vi "motionProfileTelemetry.vi"(9 "Pigeon":T2={"DeviceStatus"={"status"=FALSE, "code"=0, "source"=""}, "Device Number"=0, "Type"=352321536, "Device ID"=0, "Handle"=0, "UsageFrame"=0, "Library Path"=path ""} {"Type" items=["CAN"=352321536, "TalonSRX"=33554432]}, 10 "Alt Talon":T4={"DeviceStatus"={"status"=FALSE, "code"=0, "source"=""}, "Type"=enum."PWM", "PWM"={"PWM Channel"=enum."Invalid", "DeadBand"={"Name"="", "maxPositivePwm"=0, "minPositivePwm"=0, "centerPwm"=0, "maxNegativePwm"=0, "minNegativePwm"=0, "angularRange"=0}}, "CAN"={"Device Number"=0, "SetOutput VI Ref"=variant, "GetOutput VI Ref"=variant, "Enable VI Ref"=variant, "Disable VI Ref"=variant, "Data"=variant}, "Invert"=FALSE, "DIO PWM"={"PWM \"Enable\" Channel"=enum."Invalid", "DIOChannel"=enum."Invalid", "PWM Rate"=0.0}}, 11 "Main Talon":T4={"DeviceStatus"={"status"=FALSE, "code"=0, "source"=""}, "Type"=enum."PWM", "PWM"={"PWM Channel"=enum."Invalid", "DeadBand"={"Name"="", "maxPositivePwm"=0, "minPositivePwm"=0, "centerPwm"=0, "maxNegativePwm"=0, "minNegativePwm"=0, "angularRange"=0}}, "CAN"={"Device Number"=0, "SetOutput VI Ref"=variant, "GetOutput VI Ref"=variant, "Enable VI Ref"=variant, "Disable VI Ref"=variant, "Data"=variant}, "Invert"=FALSE, "DIO PWM"={"PWM \"Enable\" Channel"=enum."Invalid", "DIOChannel"=enum."Invalid", "PWM Rate"=0.0}}) -> ()   [LabVIEW 2018]
uses:
  <vilib>/Rock Robotics/WPI/MotorControl/WPI_MotorControlDeviceRef.ctl
  <vilib>/Rock Robotics/WPI/MotorControl/WPI_MotorControlType.ctl
  <vilib>/Rock Robotics/SystemInterfaces/DIO/FPGA_DIOPWMChannel.ctl
  <vilib>/Rock Robotics/WPI/PWM/WPI_PWMDeadband.ctl
  <vilib>/Rock Robotics/SystemInterfaces/DIO/FPGA_DIOChannel.ctl
  <vilib>/Rock Robotics/WPI/ThirdParty/Phoenix-LabVIEW/Pigeon IMU/CTRE_PigeonIMU_DeviceRef.ctl
  <vilib>/Rock Robotics/WPI/ThirdParty/Phoenix-LabVIEW/Pigeon IMU/CTRE_PigeonIMU_ConnectionType.ctl
  driveShifterEnum.ctl
  <vilib>/Rock Robotics/WPI/ThirdParty/Phoenix-LabVIEW/Pigeon IMU/CTRE_PigeonIMU_CalibrationMode.ctl
  <vilib>/Rock Robotics/WPI/ThirdParty/Phoenix-LabVIEW/Motor Controller/Get/CTRE_Phoenix_MotorController_GetVoltage.vi
  <vilib>/Rock Robotics/WPI/ThirdParty/Phoenix-LabVIEW/Motor Controller/Get/CTRE_Phoenix_MotorController_GetQuadratureData.vi
panel:
  out "driveIMUYawPitchRoll":cluster{"Yaw":dbl, "Pitch":dbl, "Roll":dbl}
  out "driveFusedHeading":T1
  in  "Calibrate IMU":bool
  in  "Reset PID":bool
  out "Percent Out":T9(graph)
  out "Motion Profile Status":T10
  out "Turn":cluster{dbl, "x-y":dbl}[](graph)
  out "Position":cluster{"x-y":dbl, i32}[](graph)
  out "Velocity":cluster{"Output":dbl, "Double":dbl}[](graph)
  out "Right Velocity":i32
  out "Right Position":i32=-2624
  out "Left Velocity":i32
  out "Left Position":i32=2620
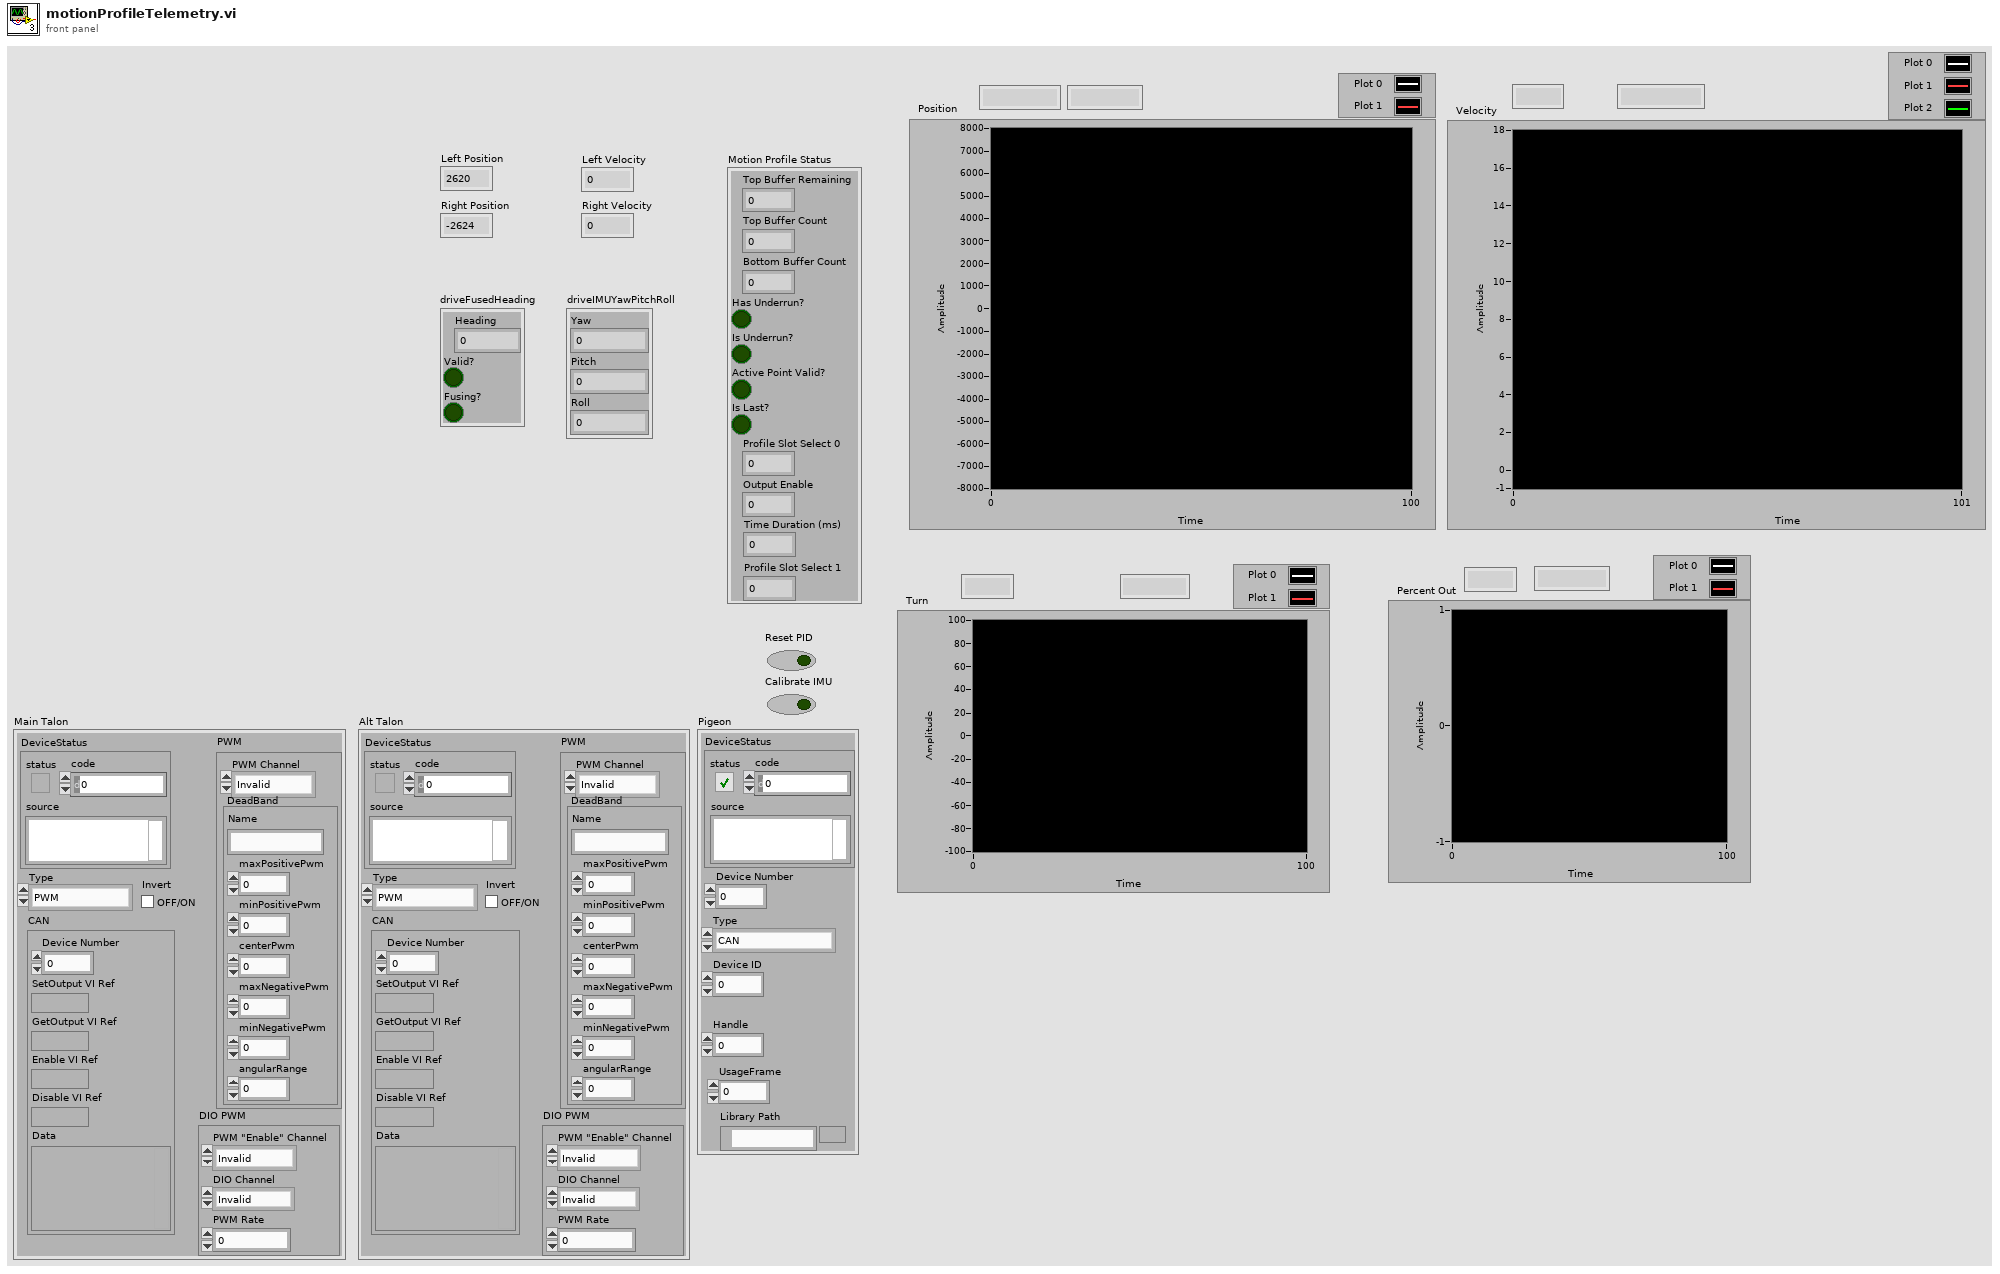
[diagram p1: front panel]
types:
  T1 = cluster{"Heading":dbl, "Valid?":bool, "Fusing?":bool}
  T2 = typedef "CTRE_PigeonIMU_DeviceRef.ctl" = cluster{"DeviceStatus":errorcluster, "Device Number":u8, "Type":T3, "Device ID":u32, "Handle":u64, "UsageFrame":u32, "Library Path":path}
  T3 = typedef "CTRE_PigeonIMU_ConnectionType.ctl" = u32
  T4 = typedef "WPI_MotorControlDeviceRef.ctl" = cluster{"DeviceStatus":errorcluster, "Type":T5, "PWM":cluster{"PWM Channel":T6, "DeadBand":T7}, "CAN":cluster{"Device Number":u8, "SetOutput VI Ref":variant, "GetOutput VI Ref":variant, "Enable VI Ref":variant, "Disable VI Ref":variant, "Data":variant}, "Invert":bool, "DIO PWM":cluster{"PWM \"Enable\" Channel":T6, "DIOChannel":T8, "PWM Rate":dbl}}
  T5 = typedef "WPI_MotorControlType.ctl" = enum16{"PWM", "CAN", "DIO PWM"}
  T6 = typedef "FPGA_DIOPWMChannel.ctl" = enum8{"PWM 0", "PWM 1", "PWM 2", "PWM 3", "PWM 4", "PWM 5", "PWM 6", "PWM 7", "PWM 8", "PWM 9", "PWM MXP 0", "PWM MXP 1", "PWM MXP 2", "PWM MXP 3", "PWM MXP 4", "PWM MXP 5", "PWM MXP 6", "PWM MXP 7", "PWM MXP 8", "PWM MXP 9", "Invalid"}
  T7 = typedef "WPI_PWMDeadband.ctl" = cluster{"Name":string, "maxPositivePwm":i32, "minPositivePwm":i32, "centerPwm":i32, "maxNegativePwm":i32, "minNegativePwm":i32, "angularRange":u16}
  T8 = typedef "FPGA_DIOChannel.ctl" = enum8{"DIO 0", "DIO 1", "DIO 2", "DIO 3", "DIO 4", "DIO 5", "DIO 6", "DIO 7", "DIO 8", "DIO 9", "DIO MXP 0", "DIO MXP 1", "DIO MXP 2", "DIO MXP 3", "DIO MXP 4", "DIO MXP 5", "DIO MXP 6", "DIO MXP 7", "DIO MXP 8", "DIO MXP 9", "DIO MXP 10", "DIO MXP 11", "DIO MXP 12", "DIO MXP 13", "DIO MXP 14", "DIO MXP 15", "SPI Port CS1", "SPI Port CS2", "SPI Port CS3", "SPI Port MISO", "SPI Port MOSI", "Invalid"}
  T9 = cluster{"Percent Output":dbl, "Percent Output":dbl}[]
  T10 = cluster{"Top Buffer Remaining":i32, "Top Buffer Count":i32, "Bottom Buffer Count":i32, "Has Underrun?":bool, "Is Underrun?":bool, "Active Point Valid?":bool, "Is Last?":bool, "Profile Slot Select 0":i32, "Output Enable":i32, "Time Duration (ms)":i32, "Profile Slot Select 1":i32}
  T11 = typedef "driveShifterEnum.ctl" = enum16{"Low", "High"}
  T12 = enum16{"Inches -> Sensor Units", "Sensor Units -> Inches"}
  T13 = typedef "CTRE_PigeonIMU_CalibrationMode.ctl" = u16
  T14 = cluster{"Percent Output":dbl, "Percent Output":dbl}
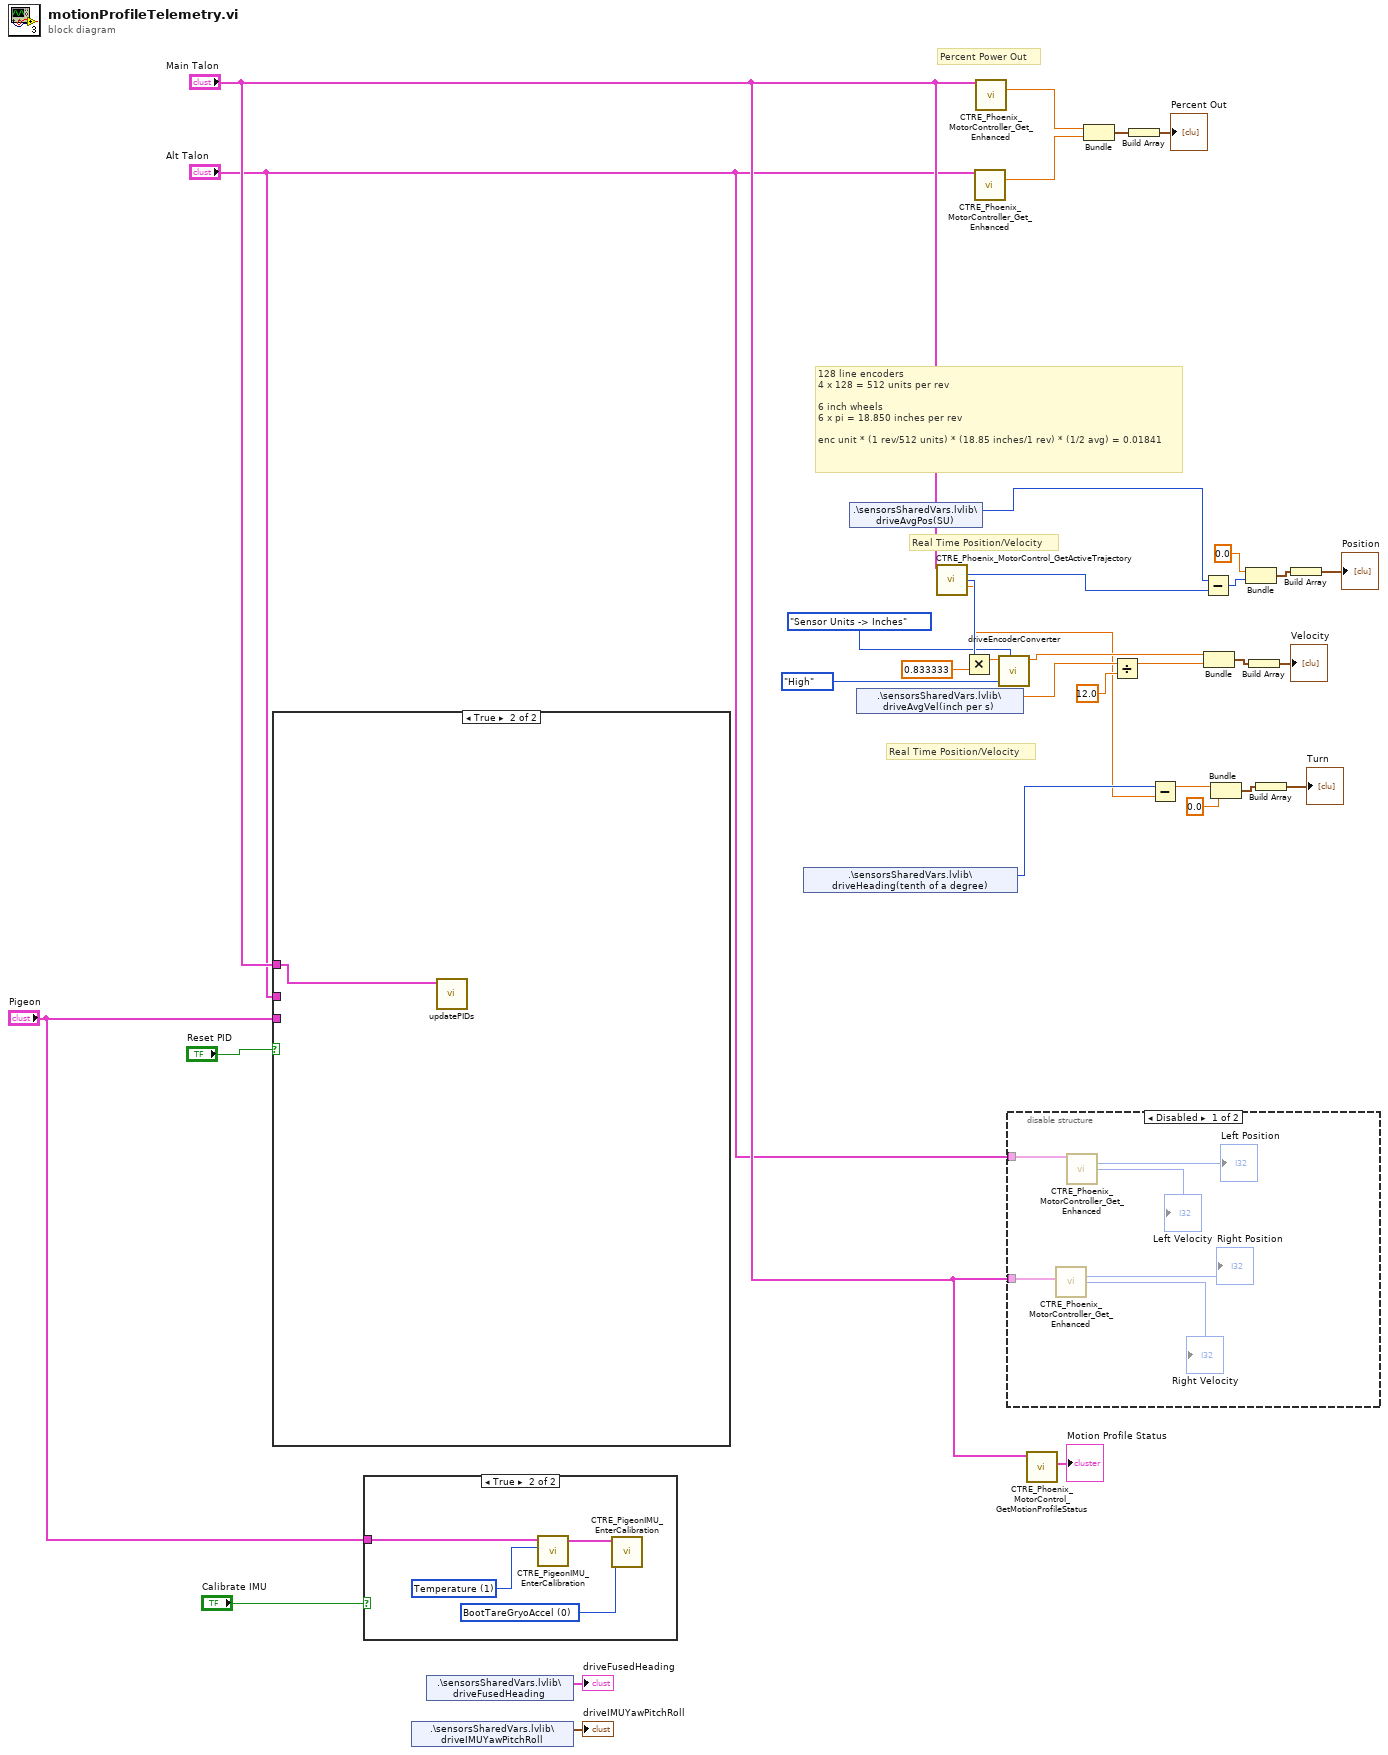
[diagram p0: block diagram]
diagram:
  # "Percent Power Out"
  # "Real Time Position/Velocity"
  # "Real Time Position/Velocity"
  # "128 line encoders\n4 x 128 = 512 units per rev\n\n6 inch wheels\n6 x pi = 18.850 inches per rev\n\nenc unit * (1 rev/512 units) * (18.85 inches/1 rev) * (1/2 avg) = 0.01841"
  n1 = case shown="True" "Reset PID" {
    tunnel: "Main Talon" -> [_ w36]
    tunnel: "Alt Talon" -> [_ _]
    tunnel: "Pigeon" -> [_ _]
    frame False {
    }
    frame True {
      n2 = call "updatePIDs.vi"("MainTalon"=w36) -> ()  [unwired: 11 in]
    }
  }
  n3 = case shown="True" "Calibrate IMU" {
    tunnel: "Pigeon" -> [_ w40]
    frame False {
    }
    frame True {
      w37 = T13 0 items=["BootTareGryoAccel"=0, "Temperature"=1, "Magnetometer12Pt"=2, "Magnetometer360"=3, "Accelerometer"=5] ("CalibrationMode")
      w39 = T13 1 items=["BootTareGryoAccel"=0, "Temperature"=1, "Magnetometer12Pt"=2, "Magnetometer360"=3, "Accelerometer"=5] ("CalibrationMode")
      n4 = call <vilib>:"CTRE_PigeonIMU_EnterCalibration.vi"("CalibrationMode"=w39, "PigeonIMUDevRef"=w40) -> ("PigeonIMUDevRef"=w38:T2)  [unwired: 8 in, 1 out]
      n5 = call <vilib>:"CTRE_PigeonIMU_EnterCalibration.vi"("CalibrationMode"=w37, "PigeonIMUDevRef"=w38) -> ()  [unwired: 8 in, 2 out]
    }
  }
  n6 = shared-variable ".\\sensorsSharedVars.lvlib\\driveIMUYawPitchRoll"() -> (→"driveIMUYawPitchRoll":cluster{"Yaw":dbl, "Pitch":dbl, "Roll":dbl})  [unwired: 1 in, 1 out]
  n7 = shared-variable ".\\sensorsSharedVars.lvlib\\driveFusedHeading"() -> (→"driveFusedHeading":T1)  [unwired: 1 in, 1 out]
  n8 = shared-variable ".\\sensorsSharedVars.lvlib\\driveHeading(tenth of a degree)"() -> (w25:i32)  [unwired: 1 in, 1 out]
  n9 = shared-variable ".\\sensorsSharedVars.lvlib\\driveAvgPos(SU)"() -> (w13:i32)  [unwired: 1 in, 1 out]
  n10 = shared-variable ".\\sensorsSharedVars.lvlib\\driveAvgVel(inch per s)"() -> (w23:dbl)  [unwired: 1 in, 1 out]
  n11 = call <vilib>:"CTRE_Phoenix_MotorControl_GetActiveTrajectory.vi"("PhoenixMotorControlDevRef"="Main Talon") -> ("Position (Sensor Units)"=w11:i32, "Velocity (Sensor Units per 100 ms)"=w22:i32, "Heading"=w9:dbl)  [unwired: 10 in, 2 out]
  n12 = Multiply(x=w22, y=0.833333) -> (x*y=w19:dbl)
  n13 = call-poly <vilib>:"CTRE_Phoenix_MotorController_Get_Enhanced.vi"("PhoenixMotorControlDevRef"="Alt Talon") -> ("Percent Output"=w2:dbl)  [unwired: 10 in, 4 out]
  n14 = call-poly <vilib>:"CTRE_Phoenix_MotorController_Get_Enhanced.vi"("PhoenixMotorControlDevRef"="Main Talon") -> ("Percent Output"=w1:dbl)  [unwired: 10 in, 4 out]
  n15 = call "driveEncoderConverter.vi"("Conversion Direction"=T12."Sensor Units -> Inches", "Gear Setting"=driveShifterEnum."High", "Input"=w19) -> ("Output"=w20:dbl)  [unwired: 8 in]
  n16 = disable-structure shown="Disabled" {
    disable-tunnel: "Main Talon" -> [w46 _]
    disable-tunnel: "Alt Talon" -> [w45 _]
    frame Disabled {
      n17 = call-poly <vilib>:"CTRE_Phoenix_MotorController_Get_Enhanced.vi"("PhoenixMotorControlDevRef"=w46) -> ("Quadrature Position"=→"Right Position":i32, "Quadrature Velocity"=→"Right Velocity":i32)  [unwired: 11 in, 2 out]
      n18 = call-poly <vilib>:"CTRE_Phoenix_MotorController_Get_Enhanced.vi"("PhoenixMotorControlDevRef"=w45) -> ("Quadrature Position"=→"Left Position":i32, "Quadrature Velocity"=→"Left Velocity":i32)  [unwired: 11 in, 2 out]
    }
    frame Enabled {
    }
  }
  n19 = call <vilib>:"CTRE_Phoenix_MotorControl_GetMotionProfileStatus.vi"("PhoenixMotorControlDevRef"="Main Talon") -> ("Motion Profile Status"=→"Motion Profile Status":T10)  [unwired: 8 in, 2 out]
  n20 = Bundle("Percent Output"=w1, "Percent Output"=w2) -> (w4:T14)  [unwired: 1 in]
  n21 = Divide(x=w23, y=12.0) -> (x/y=w17:dbl)
  n22 = Build Array(w4) -> (→"Percent Out":T9)
  n23 = Subtract(x=w25, y=w9) -> (x-y=w10:dbl)
  n24 = Subtract(x=w13, y=w11) -> (x-y=w15:i32)
  n25 = Bundle("Output"=w20, w17) -> (w28:cluster{"Output":dbl, dbl})  [unwired: 1 in]
  n26 = Bundle(w10, "x-y"=0.0) -> (w27:cluster{dbl, "x-y":dbl})  [unwired: 1 in]
  n27 = Bundle("x-y"=0.0, w15) -> (w29:cluster{"x-y":dbl, i32})  [unwired: 1 in]
  n28 = Build Array(w28) -> (→"Velocity":cluster{"Output":dbl, dbl}[])
  n29 = Build Array(w27) -> (→"Turn":cluster{dbl, "x-y":dbl}[])
  n30 = Build Array(w29) -> (→"Position":cluster{"x-y":dbl, i32}[])
